vi "set_tab_names.vi"(4 "error out 2":errorcluster, 5 "index":i32, 6 "Name":string, 7 "Tab Control":refnum<vi>) -> (0 "error out":errorcluster)   [LabVIEW 2010]
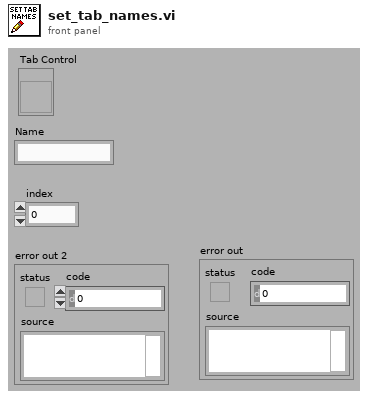
[diagram p1: front panel]
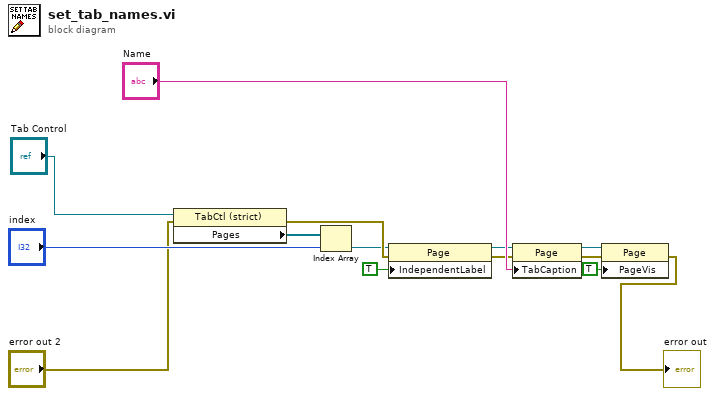
[diagram p0: block diagram]
diagram:
  n1 = property class="TabCtl (strict)"(reference="Tab Control", error in="error out 2") -> (error out=w7:errorcluster, "Pages"=w6:refnum<vi>[])  [unwired: 1 out]
  n2 = Index Array(array=w6, index="index") -> (element=w2:refnum<vi>)
  n3 = property class="Page"(reference=w2, error in=w7, "IndependentLabel"=TRUE ("Independent Label")) -> (reference out=w5:refnum<vi>, error out=w4:errorcluster)
  n4 = property class="Page"(reference=w5, error in=w4, "TabCaption"="Name") -> (reference out=w11:refnum<vi>, error out=w12:errorcluster)
  n5 = property class="Page"(reference=w11, error in=w12, "PageVis"=TRUE ("Page Visible")) -> (error out=→"error out":errorcluster)  [unwired: 1 out]
